vi "spiAccelerometerWriteByte.vi"(1 "error in (no error)":errorcluster, 2 "Data":u16 format="%.0b", 3 "Address":u16 format="%.0b") -> (0 "error out":errorcluster)   [LabVIEW 2012]
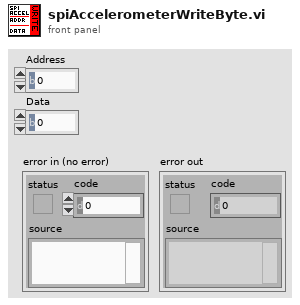
[diagram p1: front panel]
types:
  T1 = typedef "WPI_SPIDevRef.ctl" = cluster{"DevStatus":errorcluster}
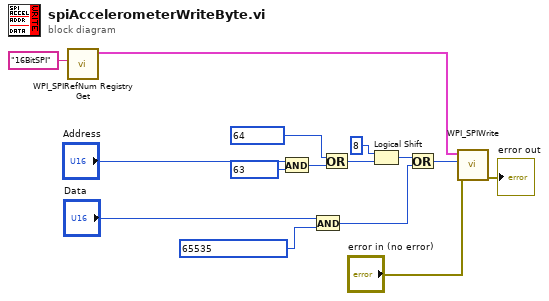
[diagram p0: block diagram]
diagram:
  n1 = call <vilib>:"WPI_SPIRefNum Registry Get.vi"("refnum name"="16BitSPI") -> ("SPIDevRef"=w5:T1)  [unwired: 9 in, 1 out]
  n2 = And(x="Address", y=u16 63) -> (x .and. y?=w14:u16)
  n3 = And(x="Data", y=u16 65535) -> (x .and. y?=w6:u16)
  n4 = Or(x=u16 64, y=w14) -> (x .or. y?=w9:u16)
  n5 = Logical Shift(y=i16 8, x=w9) -> (x << y=w10:u16)
  n6 = Or(x=w10, y=w6) -> (x .or. y?=w7:u16)
  n7 = call <vilib>:"WPI_SPIWrite.vi"("error in (no error)"="error in (no error)", "Data To Send"=w7, "SPIDevRef"=w5) -> ("error out"=→"error out":errorcluster)  [unwired: 7 in, 1 out]
